vi "WFDC Get Current Image.vi"(0 "IDS Camera Notifier Name":string, 11 "Error":errorcluster, 13 "Frames":u16) -> (4 "IDS Camera Notifier Name (Dup)":string, 8 "Image - U16":u16[][](array[numeric]), 15 "Error":errorcluster)   [LabVIEW 2016]
uses:
  Device Library/Cameras/IDS/IDS Controls/IDS IMAQ Key Info.ctl
  Device Library/Cameras/IDS/IDS Controls/IDS Actions.ctl
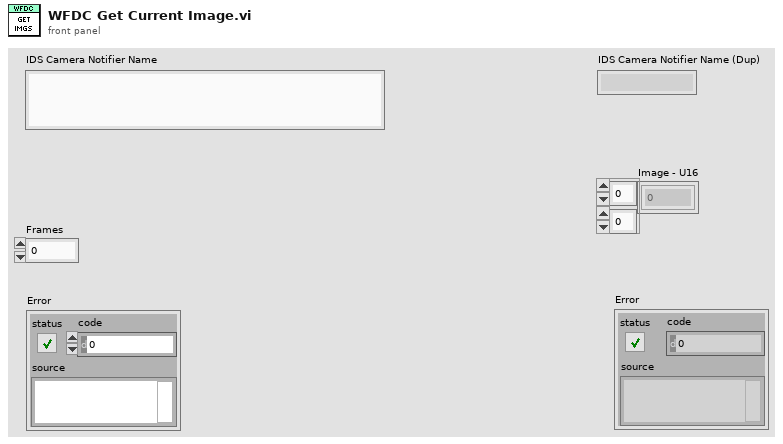
[diagram p1: front panel]
types:
  T1 = typedef "IDS Actions.ctl" = enum16{"Error Check", "Initialize", "Preview", "Record", "Abort", "Record Settings", "Set Parameter", "Get Parameter", "Set ROI", "Get ROI", "Status", "Quit"}
  T2 = typedef "IDS IMAQ Key Info.ctl" = cluster{"Frame":u32, "Sensor Height":i32, "Sensor Width":i32, "ROI Height":i32, "ROI Width":i32, "ROI Enable?":bool, "Bit per Pixel":u8}
  T3 = typedef "IMAQ Image.ctl" = refnum<image>
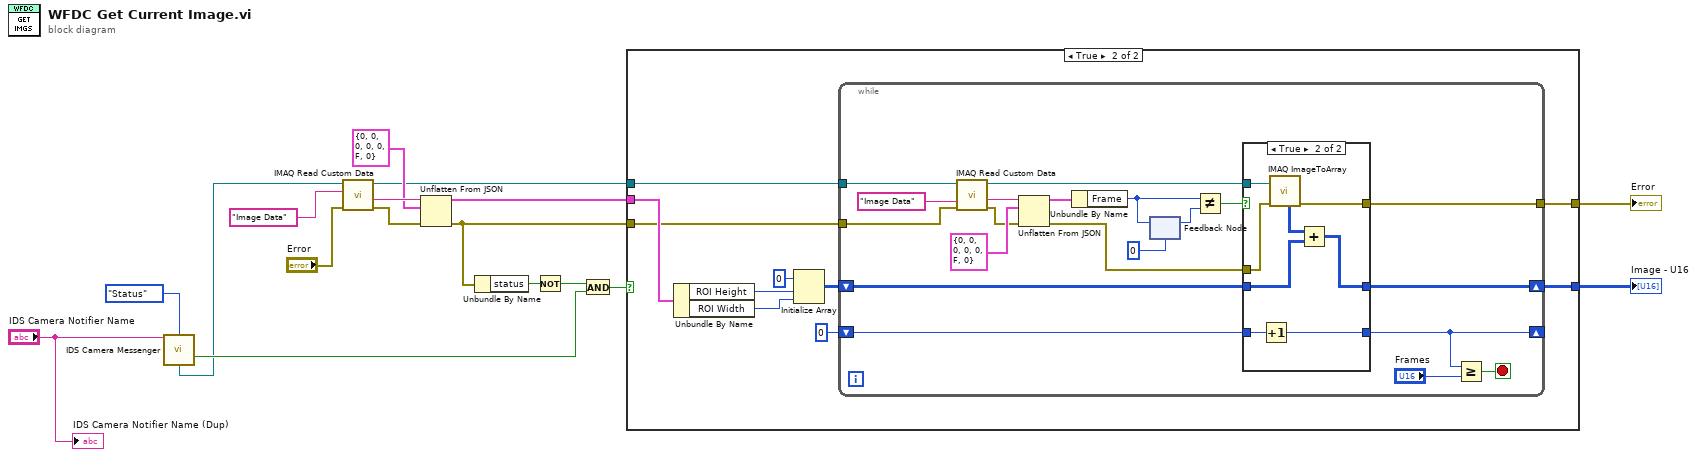
[diagram p0: block diagram]
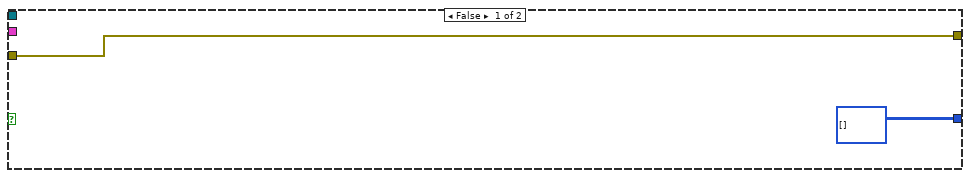
[diagram p2: hidden frame]
diagram:
  n1 = call "IDS Camera Messenger.vi"("Notifier Name"="IDS Camera Notifier Name", "IDS Actions"=IDS_Actions."Status") -> ("Running?"=w7:bool, "Image Ref"=w2:T3)  [unwired: 8 in, 4 out]
  n2 = call "IMAQ Read Custom Data"("error in (no error)"="Error", "Key"="Image Data", "Image"=w2) -> ("error out"=w10:errorcluster, "Custom Data Out"=w16:string, "Image (duplicate)"=w13:T3)  [unwired: 6 in]
  n3 = Unflatten From JSON(JSON string=w16, type and defaults=T2 {"Frame"=0, "Sensor Height"=0, "Sensor Width"=0, "ROI Height"=0, "ROI Width"=0, "ROI Enable?"=FALSE, "Bit per Pixel"=0} ("IDS IMAQ Key Info"), error in (no error)=w10) -> (value=w14:T2, error out=w5:errorcluster)  [unwired: 4 in]
  n4 = Unbundle By Name(w5) -> ("status"=w9:bool)
  n5 = Not(x=w9) -> (.not. x?=w8:bool)
  n6 = And(x=w8, y=w7) -> (x .and. y?=w6:bool)
  n7 = case shown="True" w6 {
    tunnel: w14 -> [_ w28]
    tunnel: w13 -> [_ w23]
    tunnel: w5 -> [w19 w22]
    tunnel: [w19 w21] -> w4
    tunnel: [u16[][] [] w20] -> w3
    frame False {
    }
    frame True {
      n8 = Unbundle By Name(w28) -> ("ROI Height"=w27:i32, "ROI Width"=w26:i32)
      n9 = Initialize Array(u16 0 ("element"), w27, w26) -> (w24:u16[][])
      n10 = while {
        shift-right: [w37] -> _
        shift-left: u16 0 -> [w38]
        shift-right: [w35] -> w20
        shift-left: w24 -> [w39]
        tunnel: w23 -> [w46]
        tunnel: w22 -> [w33]
        tunnel: [w30] -> w21
        stop <- w36 stop-if-true
        n11 = call "IMAQ Read Custom Data"("error in (no error)"=w33, "Key"="Image Data", "Image"=w46) -> ("error out"=w32:errorcluster, "Custom Data Out"=w48:string, "Image (duplicate)"=w40:T3)  [unwired: 6 in]
        n12 = Unflatten From JSON(JSON string=w48, type and defaults=T2 {"Frame"=0, "Sensor Height"=0, "Sensor Width"=0, "ROI Height"=0, "ROI Width"=0, "ROI Enable?"=FALSE, "Bit per Pixel"=0} ("IDS IMAQ Key Info"), error in (no error)=w32) -> (value=w45:T2, error out=w31:errorcluster)  [unwired: 4 in]
        n13 = Unbundle By Name(w45) -> ("Frame"=w43:u32)
        n14 = feedback-in #1(w43) -> ()
        n15 = feedback #1(u32 0) -> (w42:u32)
        n16 = Not Equal?(x=w43, y=w42) -> (x != y?=w41:bool)
        n17 = case shown="True" w41 {
          tunnel: w40 -> [_ w58]
          tunnel: w39 -> [w52 w57]
          tunnel: w38 -> [w51 w60]
          tunnel: [w51 w59] -> w37
          tunnel: [w52 w56] -> w35
          tunnel: w31 -> [w50 w55]
          tunnel: [w50 w54] -> w30
          frame False {
          }
          frame True {
            n18 = Increment(x=w60) -> (x+1=w59:u16)
            n19 = call "IMAQ ImageToArray"("error in (no error)"=w55, "Image"=w58) -> ("Image Pixels (U16)"=w53:u16[][], "error out"=w54:errorcluster)  [unwired: 2 in, 3 out]
            n20 = Add(x=w53, y=w57) -> (x+y=w56:u16[][])
          }
        }
        n21 = Greater Or Equal?(x=w37, y="Frames") -> (x >= y?=w36:bool)
      }
    }
  }
  "Error" <- w4
  "Image - U16" <- w3
  "IDS Camera Notifier Name (Dup)" <- "IDS Camera Notifier Name"
